vi "add_uint8.vi"   [LabVIEW 2015]
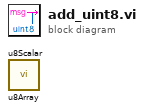
[diagram p0: block diagram]
diagram:
  n1 = call "u8Array.vi"() -> ()  [unwired: 5 in, 1 out]
  n2 = call "u8Scalar.vi"() -> ()  [unwired: 5 in, 1 out]
